vi "Edit Labels.vi"(6 "Variant in":variant, 7 "Shift Pressed?":bool, 8 "error in (no error)":errorcluster, 10 "QD Combo Box Ref":refnum<vi>, 11 "QD Launch VI Ref":refnum<vi>) -> (0 "error out":errorcluster, 4 "Variant out":variant)   [LabVIEW 2015]
doc: "Removes the selected block diagram object(s) and any wires and constants connected to the selected object(s), and connects wires of identical data types that were wired to the inputs and outputs of the deleted object(s).\n\nDefault Shortcut - [R]"
uses:
  <vilib>/Utility/traverseref.llb/TRef TravTarget.ctl
  <vilib>/Utility/traverseref.llb/VI Scripting - Traverse.lvlib
panel:
  in  "Undo Name":string="Quick Drop Remove"
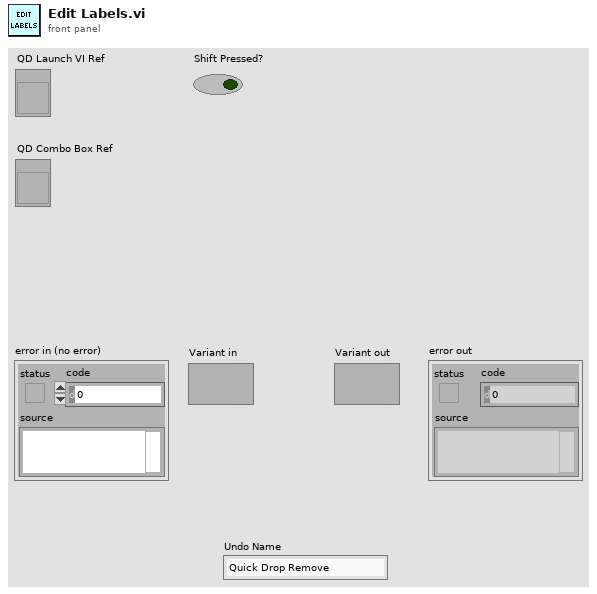
[diagram p1: front panel]
types:
  T1 = typedef "TRef TravTarget.ctl" = enum16{"FP", "BD", "Other"}
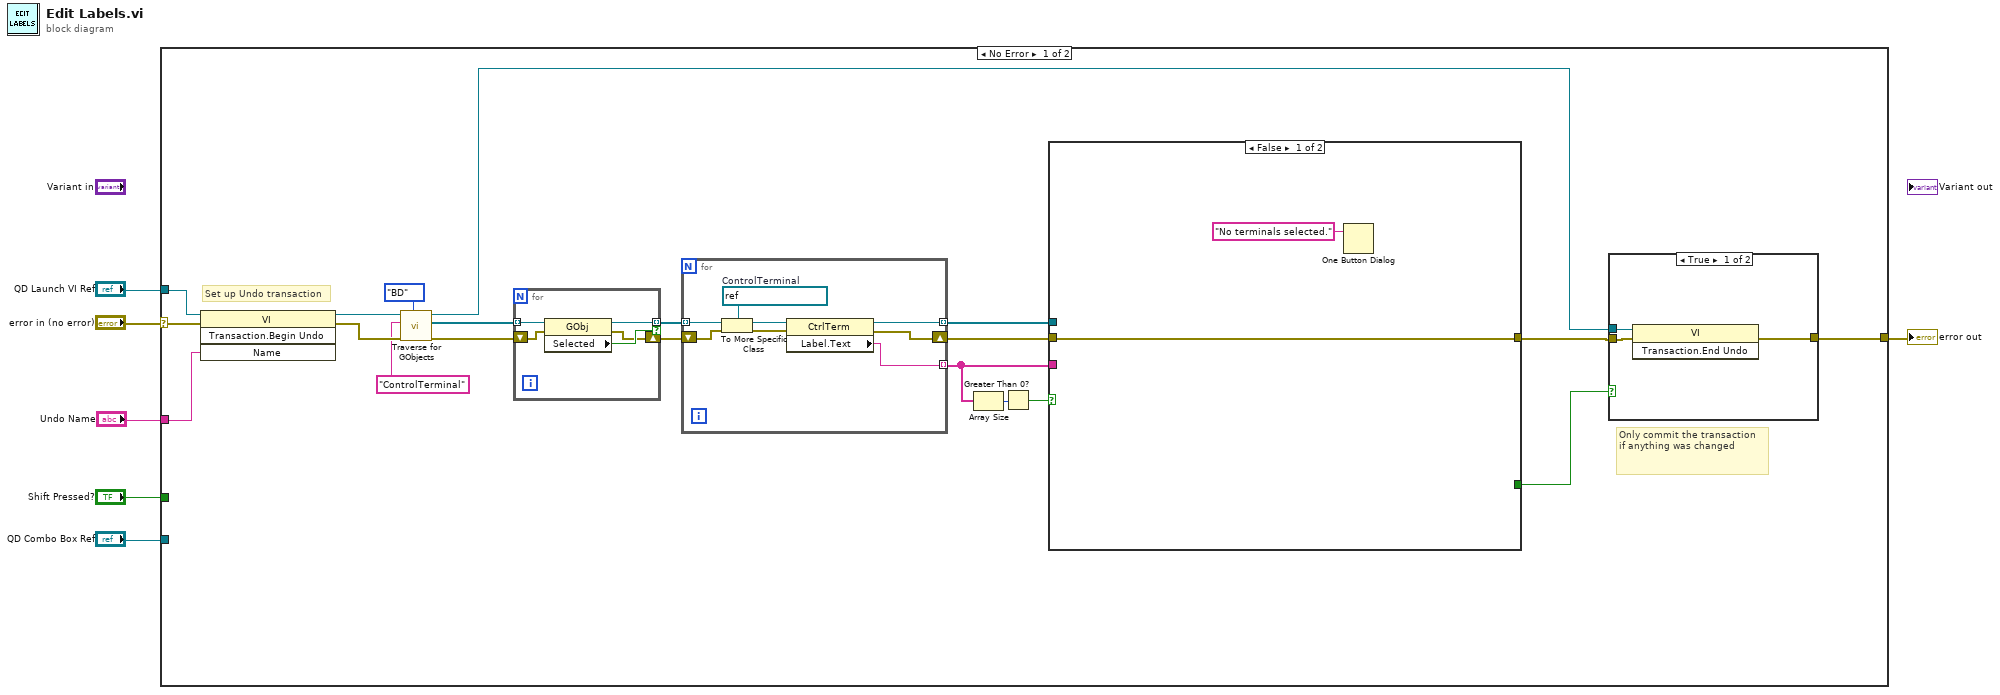
[diagram p0: block diagram]
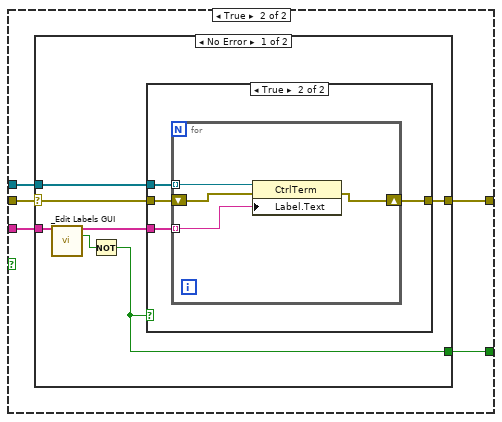
[diagram p2: hidden frame]
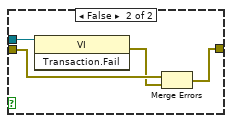
[diagram p5: hidden frame]
diagram:
  n1 = case shown="No Error" "error in (no error)" {
    selector: "error in (no error)" -> [w26 w71]
    tunnel: [w24 w71] -> w5
    tunnel: "QD Launch VI Ref" -> [w25 _]
    tunnel: "Shift Pressed?" -> [_ _]
    tunnel: "QD Combo Box Ref" -> [_ _]
    tunnel: "Undo Name" -> [w23 _]
    frame No Error {
      # "Set up Undo transaction"
      # "Only commit the transaction\nif anything was changed"
      n2 = invoke class="VI" method="Transaction.Begin Undo"(reference=w25, error in=w26, "Name"=w23) -> (reference out=w21:refnum<vi>, error out=w20:errorcluster)  [unwired: 1 in, 2 out]
      n3 = call <vilib>:"Traverse for GObjects.vi"("Traverse Target"=TRef_TravTarget."BD", "error in (no error)"=w20, "Class Name"="ControlTerminal", "VI Refnum"=w21) -> ("error out"=w11:errorcluster, "References"=w10:refnum<vi>[], "dup VI Refnum"=w12:refnum<vi>)  [unwired: 4 in, 1 out]
      n4 = for {
        tunnel: w10 -> [w55] mode=indexing
        tunnel: [w54] -> w19 mode=indexing if=w53
        shift-right: [w51] -> w18
        shift-left: w11 -> [w52]
        n5 = property class="GObj"(reference=w55, error in=w52) -> (reference out=w54:refnum<vi>, error out=w51:errorcluster, "Selected"=w53:bool)
      }
      n6 = for {
        tunnel: w19 -> [w63] mode=indexing
        shift-right: [w57] -> w16
        shift-left: w18 -> [w60]
        tunnel: [w58] -> w17 mode=indexing
        tunnel: [w56] -> w9 mode=indexing
        w62 = refnum<vi> refnum  # ControlTerminal
        n7 = To More Specific Class(target class=w62, reference=w63, error in=w60) -> (specific class reference=w61:refnum<vi>, error out=w59:errorcluster)
        n8 = property class="CtrlTerm"(reference=w61, error in=w59) -> (reference out=w58:refnum<vi>, error out=w57:errorcluster, "Label.Text"=w56:string)
      }
      n9 = Array Size(array=w9) -> (size(s)=w8:i32)
      n10 = Greater Than 0?(x=w8) -> (x > 0?=w7:bool)
      n11 = case shown="False" w7 {
        tunnel: w17 -> [_ w33]
        tunnel: w9 -> [_ w32]
        tunnel: w16 -> [w28 w31]
        tunnel: [w28 w30] -> w15
        tunnel: [_ w29] -> w14
        frame False {
          n12 = One Button Dialog(message="No terminals selected.") -> ()  [unwired: 1 in, 1 out]
        }
        frame True {
          n13 = case shown="No Error" w31 {
            selector: w31 -> [w36 w50]
            tunnel: w33 -> [w40 _]
            tunnel: [w39 w50] -> w30
            tunnel: w32 -> [w38 _]
            tunnel: [w34 _] -> w29
            frame No Error {
              n14 = call <resource>:"_Edit Labels GUI.vi"("labels in"=w38) -> ("labels out"=w37:string[], "canceled"=w35:bool)  [unwired: 13 in]
              n15 = Not(x=w35) -> (.not. x?=w34:bool)
              n16 = case shown="True" w34 {
                tunnel: w40 -> [_ w45]
                tunnel: w36 -> [w41 w44]
                tunnel: [w41 w43] -> w39
                tunnel: w37 -> [_ w42]
                frame False {
                }
                frame True {
                  n17 = for {
                    tunnel: w45 -> [w49] mode=indexing
                    shift-right: [w47] -> w43
                    shift-left: w44 -> [w48]
                    tunnel: w42 -> [w46] mode=indexing
                    n18 = property class="CtrlTerm"(reference=w49, error in=w48, "Label.Text"=w46) -> (error out=w47:errorcluster)  [unwired: 1 out]
                  }
                }
              }
            }
            frame Error {
            }
          }
        }
      }
      n19 = case shown="True" w14 {
        tunnel: w12 -> [w65 w70]
        tunnel: [w66 w67] -> w24
        tunnel: w15 -> [w64 w69]
        frame True {
          n20 = invoke class="VI" method="Transaction.End Undo"(reference=w65, error in=w64) -> (error out=w66:errorcluster)  [unwired: 1 in, 2 out]
        }
        frame False {
          n21 = invoke class="VI" method="Transaction.Fail"(reference=w70) -> (error out=w68:errorcluster)  [unwired: 2 in, 2 out]
          n22 = Merge Errors(w69, w68) -> (w67:errorcluster)
        }
      }
    }
    frame Error {
    }
  }
  "error out" <- w5
